vi "Front_Panel.vi"() -> ()   [LabVIEW 2020]
panel:
  in  "Tab Control":enum32{"Page 1", "Page 2", "Page 3"}(tab)
  in  "On/Off":bool
  out "Angle:":dbl
  out "Gain:":dbl
  in  "Position":dbl(slide) scale=0.0..10.0
  out "Waveform Graph":dbl[](graph)
  in  "On/Off 2":bool
  out "Angle:  2":dbl
  out "Gain:  2":dbl
  in  "Position 2":dbl(slide) scale=0.0..10.0
  out "Waveform Graph 2":dbl[](graph)
  out "On/Off 3":bool
  out "Band Width:":dbl
  out "Frequency:":dbl
  out "IP Address:":string
  out "On/Off":bool
  out "Band Width:":dbl
  out "Frequency:":dbl
  out "IP Address:":string
  out "Source to :":string
  out "PILOT:":string
  # "RX PANEL"
  # "Beam"
  # "TX PANEL"
  # "Beam"
  # "CIS PANEL"
  # "TX Baseband"
  # "RX Baseband"
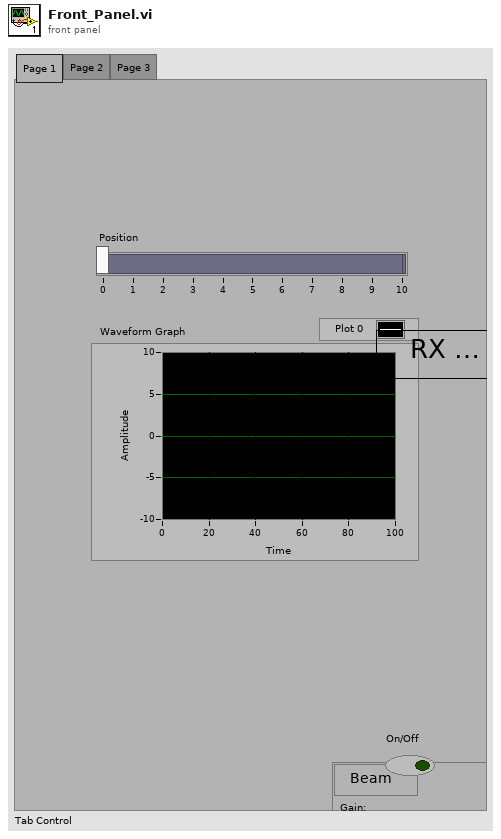
[diagram p1: front panel]
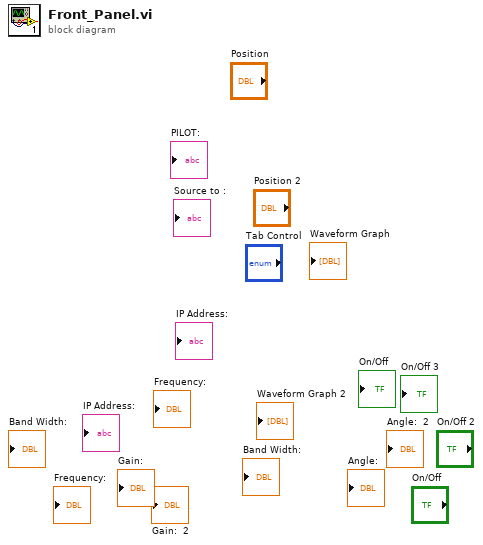
[diagram p0: block diagram]
diagram:
